vi "Get and Initialize GMLAN PID Channel References.vi"(8 "error in (no error)":errorcluster, 10 "PIDs":T3[](array[typedef]) {"Signals"."Byte Order" items=["Little Endian", "Big Endian"]; "Signals"."Data Type" items=["Signed", "Unsigned", "IEEE Float"]}, 11 "DPIDs":T1[](array[typedef])) -> (0 "error out":errorcluster, 3 "Lookup Table":variant)   [LabVIEW 2013, in "Diagnostics Addon Engine.lvlib"]
uses:
  Diagnostics Addon Engine.lvlib
  Shared/DIDPID Parameters.ctl
  Shared/DIDPID Signal Parameters.ctl
  Shared/DPID Parameters.ctl
  Shared/DPID Periodic Rate.ctl
  DPID Lookup Cluster.ctl
  DPID Lookup PID Information.ctl
  Datatable Lookup Positions.ctl
  Shared/Diagnostics Addon Shared.lvlib
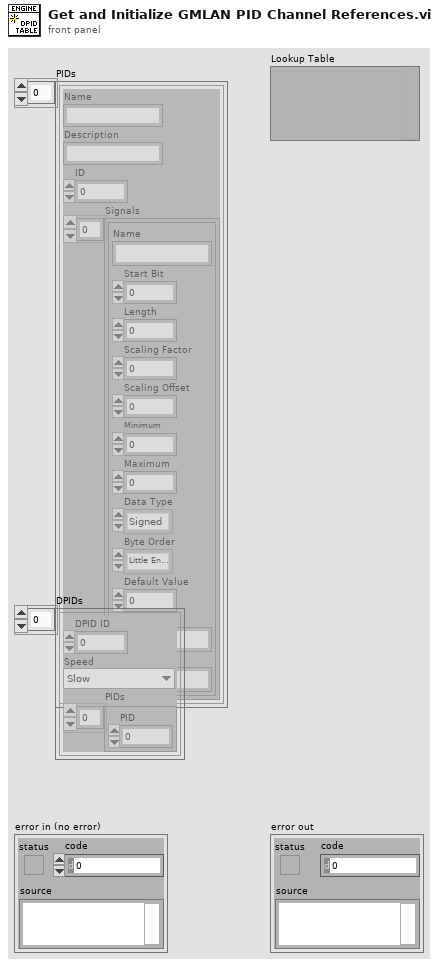
[diagram p1: front panel]
types:
  T1 = typedef "Diagnostics Addon Shared.lvlib/DPID Parameters.ctl" = cluster{"DPID ID":u8, "Speed":T2, "PIDs":u16[]}
  T2 = typedef "Diagnostics Addon Shared.lvlib/DPID Periodic Rate.ctl" = enum16{"Slow", "Medium", "Fast"}
  T3 = typedef "Diagnostics Addon Shared.lvlib/DIDPID Parameters.ctl" = cluster{"Name":string, "Description":string, "ID":u16, "Signals":T4[]}
  T4 = typedef "Diagnostics Addon Shared.lvlib/DIDPID Signal Parameters.ctl" = cluster{"Name":string, "Start Bit":u8, "Length":u8, "Scaling Factor":dbl, "Scaling Offset":dbl, "Minimum":dbl, "Maximum":dbl, "Data Type":u32, "Byte Order":u32, "Default Value":dbl, "Units":string, "Description":string}
  T5 = typedef "Diagnostics Addon Engine.lvlib/DPID Lookup Cluster.ctl" = cluster{"PID Info":T6, "Datatable Lookup":T7, "Conversion":refnum<k21>}
  T6 = typedef "Diagnostics Addon Engine.lvlib/DPID Lookup PID Information.ctl" = cluster{"PID":u16, "Frame Length":u8}
  T7 = typedef "Diagnostics Addon Engine.lvlib/Datatable Lookup Positions.ctl" = cluster{"Offset":i32, "Length":i32}
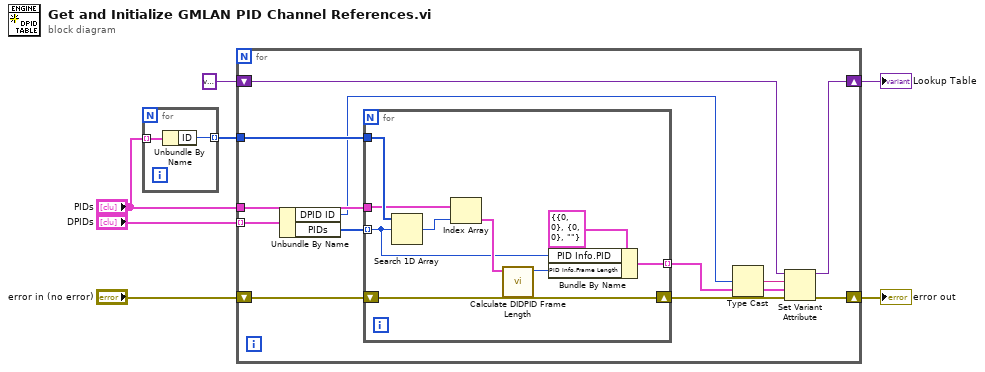
[diagram p0: block diagram]
diagram:
  n1 = for {
    tunnel: "PIDs" -> [w9] mode=indexing
    tunnel: [w8] -> w3 mode=indexing
    n2 = Unbundle By Name(w9) -> ("ID"=w8:u16)
  }
  n3 = for {
    tunnel: "DPIDs" -> [w21] mode=indexing
    tunnel: w3 -> [w20]
    tunnel: "PIDs" -> [w18]
    shift-right: [w11] -> w5
    shift-left: variant -> [w17]
    shift-right: [w12] -> w1
    shift-left: "error in (no error)" -> [w15]
    n4 = Unbundle By Name(w21) -> ("DPID ID"=w16:u8, "PIDs"=w19:u16[])
    n5 = for {
      tunnel: w20 -> [w30]
      tunnel: w19 -> [w25] mode=indexing
      tunnel: w18 -> [w29]
      shift-right: [w26] -> w14
      shift-left: w15 -> [w26]
      tunnel: [w23] -> w10 mode=indexing
      n6 = Search 1D Array(1D array=w30, element=w25) -> (index of element=w28:i32)  [unwired: 1 in]
      n7 = Index Array(array=w29, index=w28) -> (element=w27:T3)
      n8 = call "Calculate DIDPID Frame Length.vi"("PID In"=w27) -> ("Frame Length"=w24:u8)  [unwired: 10 in]
      n9 = Bundle By Name(cluster=T5 {"PID Info"={"PID"=0, "Frame Length"=0}, "Datatable Lookup"={"Offset"=0, "Length"=0}, "Conversion"=""} ("Cluster"), "PID Info.PID"=w25, "PID Info.Frame Length"=w24) -> (w23:T5)
    }
    n10 = Type Cast(x=w16) -> (*(type *) &x=w13:string)  [unwired: 1 in]
    n11 = Set Variant Attribute(Variant=w17, name=w13, value=w10, error in=w14) -> (Variant out=w11:variant, error out=w12:errorcluster)  [unwired: 1 out]
  }
  "error out" <- w1
  "Lookup Table" <- w5
